vi "Decompose LabVIEW Object - Interface - Returns No Error.vi"() -> ()   [LabVIEW 2020, in "Composition.Tests.lvlib"]
uses:
  Composition.Tests.lvlib
  IDisposable/IDisposable.lvclass
  <vilib>/addons/_JKI Toolkits/Caraya/classes/Assert/Assert Not Error.vi
  Composition/Composition.lvlib
  <vilib>/addons/_JKI Toolkits/Caraya/classes/Test/Test.lvclass
  <vilib>/addons/_JKI Toolkits/Caraya/classes/Assert/Assert.lvclass
panel:
  out "error out":errorcluster
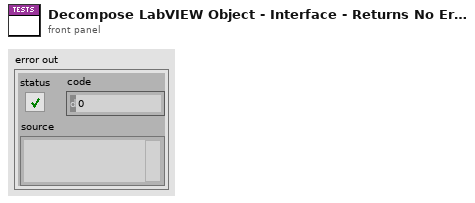
[diagram p1: front panel]
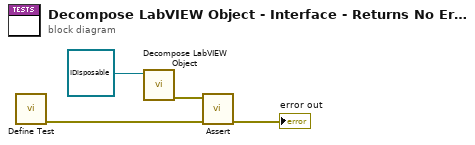
[diagram p0: block diagram]
diagram:
  n1 = call <vilib>:"Define Test.vi"() -> ("error out"=w1:errorcluster)  [unwired: 11 in]
  n2 = call "Decompose LabVIEW Object.vi"("LabVIEW Object"=refnum<class "IDisposable.lvclass"> refnum ("Reflection.Tests.lvlib:String.lvclass")) -> ("error out"=w2:errorcluster)  [unwired: 7 in, 3 out]
  n3 = call-poly <vilib>:"Assert.vi"("error in (no error)"=w1, "Not Error?"=w2) -> ("error out"=→"error out":errorcluster)  [unwired: 9 in]
